vi "Write Command Processor State.vi"(8 "error in (no error)":errorcluster, 10 "Command Processor State":T1 {"Commands Behind" scale=0.0..10.0; "Queued Commands" scale=0.0..100.0}, 11 "Command Processor in":refnum<class "Command Processor Actor.lvclass">) -> (0 "error out":errorcluster, 3 "Command Processor out":refnum<class "Command Processor Actor.lvclass">)   [LabVIEW 2014, in "Robot Actor Framework.lvlib" / "Command Processor Actor.lvlib" / "Command Processor Actor.lvclass"]
uses:
  Command Processor Actor.lvclass
  Command Processor State.ctl
  Command Processor States.ctl
  Command Actor/Command Actor Class/Command State.ctl
  Command Actor/Command Actor Class/Command States.ctl
  <vilib>/ActorFramework/Message Enqueuer/Message Priority.ctl
  <vilib>/ActorFramework/Actor/Actor.lvclass/Actor.ctl
  Command Processor Actor.lvclass/Command Processor Actor.ctl
  System Actor/System Actor Messages/Updated Command Processor Status Msg/Updated Command Processor Status Msg.lvclass/Updated Command Processor Status Msg.ctl
  <vilib>/ActorFramework/Message Enqueuer/Message Enqueuer.lvclass/Message Enqueuer.ctl
  <vilib>/ActorFramework/Message Enqueuer/Enqueue.vi
  <vilib>/ActorFramework/Message Priority Queue/Priority Enqueue.vi
  System Actor/System Actor Messages/Updated Command Processor Status Msg/Updated Command Processor Status Msg.lvclass
  <vilib>/ActorFramework/Actor/Actor.lvclass
  <vilib>/ActorFramework/Message Enqueuer/Message Enqueuer.lvclass
  Command Actor/Command Actor Class/Command Actor.lvclass
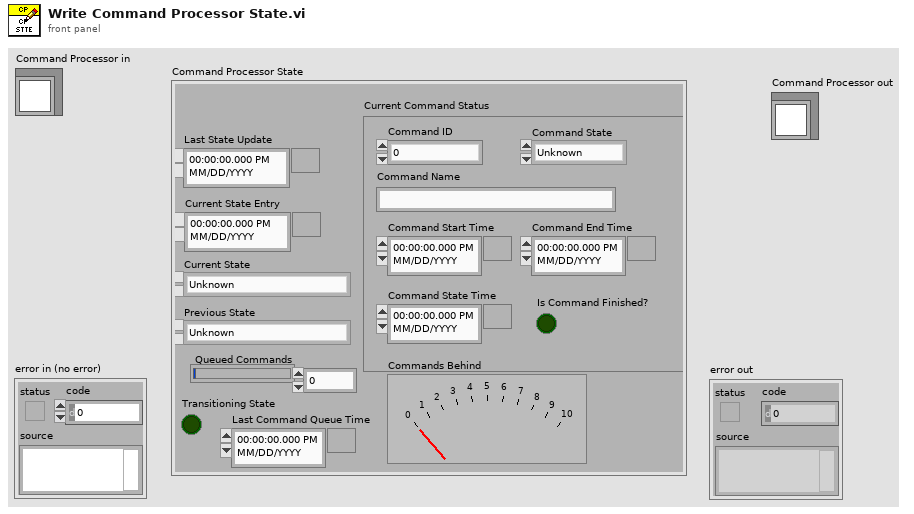
[diagram p1: front panel]
types:
  T1 = typedef "Robot Actor Framework.lvlib/Command Processor Actor.lvlib/Command Processor Actor.lvclass/Command Processor State.ctl" = cluster{"Current State":T2, "Last State Update":timestamp, "Queued Commands":u32, "Current Command Status":T3, "Previous State":T2, "Current State Entry":timestamp, "Transitioning State":bool, "Commands Behind":dbl, "Last Command Queue Time":timestamp}
  T2 = typedef "Robot Actor Framework.lvlib/Command Processor Actor.lvlib/Command Processor Actor.lvclass/Command Processor States.ctl" = enum16{"Unknown", "No Command", "Running Command", "Starting Command", "Stopping Command", "Finishing Command"}
  T3 = typedef "Robot Actor Framework.lvlib/Command Actor.lvlib/Command Actor.lvclass/Command State.ctl" = cluster{"Command Name":string, "Command Start Time":timestamp, "Command End Time":timestamp, "Is Command Finished?":bool, "Command ID":u32, "Command State":T4, "Command State Time":timestamp}
  T4 = typedef "Robot Actor Framework.lvlib/Command Actor.lvlib/Command Actor.lvclass/Command States.ctl" = enum16{"Unknown", "Started", "Stopped", "Finished"}
  T5 = typedef "Actor Framework.lvlib/Message Enqueuer.lvclass/Message Priority.ctl" = enum16{"Low", "Normal", "High"}
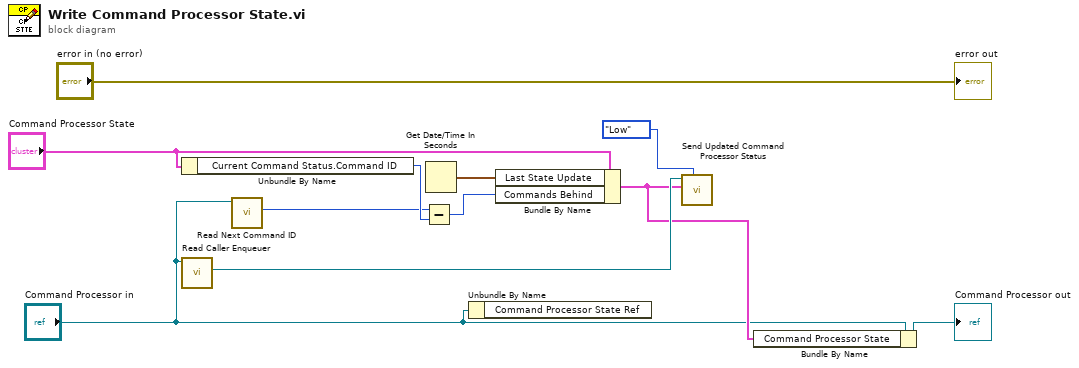
[diagram p0: block diagram]
diagram:
  n1 = Unbundle By Name("Command Processor State") -> ("Current Command Status.Command ID"=w7:u32)
  n2 = call <vilib>:"Read Caller Enqueuer.vi"("Actor"="Command Processor in") -> ("Caller Enqueuer"=w9:refnum<class "Message Enqueuer.lvclass">)  [unwired: 10 in]
  n3 = call-dynamic "Read Next Command ID.vi"("Command Processor Actor in"="Command Processor in") -> ("Next Command ID"=w4:u32)  [unwired: 8 in, 2 out]
  n4 = Subtract(x=w4, y=w7) -> (x-y=w6:u32)
  n5 = Get Date/Time In Seconds() -> (seconds since 1Jan1904=w8:timestamp)
  n6 = Unbundle By Name("Command Processor in") -> ()  [unwired: 1 out]
  n7 = Bundle By Name(cluster="Command Processor State", "Last State Update"=w8, "Commands Behind"=w6) -> (w2:T1)
  n8 = call "Send Updated Command Processor Status.vi"("Message Priority (Normal)"=Message_Priority."Low", "Command Processor Status"=w2, "Message Enqueuer"=w9) -> ()  [unwired: 7 in, 2 out]
  n9 = Bundle By Name(cluster="Command Processor in", "Command Processor State"=w2) -> (→"Command Processor out":refnum<class "Command Processor Actor.lvclass">)
  "error out" <- "error in (no error)"
